vi "Launch On-Grid Optimization.vi"(8 "error in":errorcluster, 11 "SCADA in":refnum<class "EMS.lvclass">) -> (0 "error out":errorcluster, 3 "SCADA out":refnum<class "EMS.lvclass">)   [LabVIEW 2018, in "EMS Core.lvlib" / "EMS.lvclass"]
uses:
  EMS.lvclass
  C:/Users/Administrator/Desktop/LabVIEW EMS/EMS Generic Actor/EMS Generic/EMS Generic.lvclass
  C:/Program Files (x86)/National Instruments/LabVIEW 2018/vi.lib/ActorFramework/Actor/Actor.lvclass
  Optimization/On-Grid Actor/On-Grid/On-Grid.lvclass
  C:/Users/Administrator/Desktop/LabVIEW EMS/Device Communication and Control Abstract Actor/Device Communication and Control Abstract/Device Communication and Control Abstract.lvclass
  C:/Users/Administrator/Desktop/LabVIEW EMS/Optimization/Generic Optimization Actor/Generic Optimization/Generic Optimization.lvclass
  EMS Messages/Unintentional Island Occurence Msg/Unintentional Island Occurence Msg.lvclass
  C:/Users/Administrator/Desktop/LabVIEW EMS/Optimization/Generic Optimization Actor/Generic Optimization Messages/Operation Complete Msg/Operation Complete Msg.lvclass
  Optimization/Generic Optimization Actor/Generic Optimization/Generic Optimization.lvclass/Generic Optimization.ctl
  EMS.lvclass/EMS.ctl
  <vilib>/ActorFramework/Actor/Actor.lvclass
  Optimization/Generic Optimization Actor/Generic Optimization/Generic Optimization.lvclass
  Global Variables/Global Variables.vi
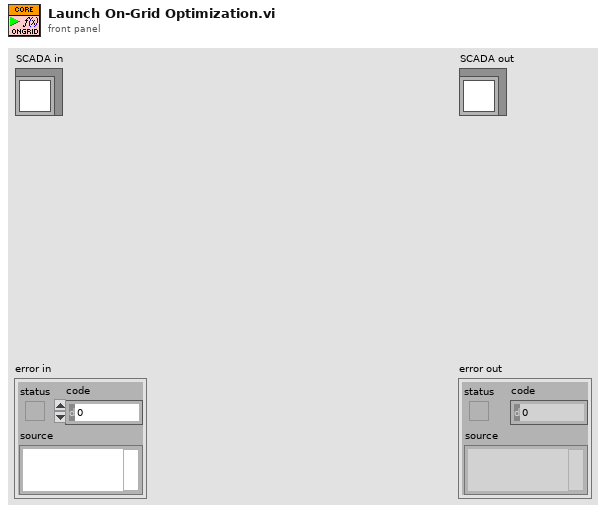
[diagram p1: front panel]
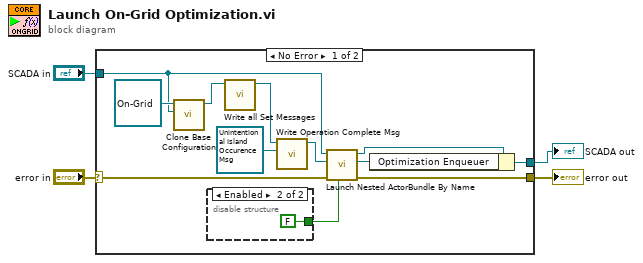
[diagram p0: block diagram]
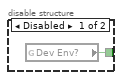
[diagram p2: hidden frame]
diagram:
  n1 = case shown="No Error" "error in" {
    selector: "error in" -> [w9 w20]
    tunnel: [w15 w20] -> w3
    tunnel: [w14 w19] -> w1
    tunnel: "SCADA in" -> [w6 w19]
    frame No Error {
      n2 = call-dynamic "Clone Base Configuration.vi"("Source Object"=w6, "Target Object in"=refnum<class "On-Grid.lvclass"> refnum ("On-Grid Actor.lvlib:On-Grid.lvclass")) -> ("Target Object out"=w7:refnum<class "On-Grid.lvclass">)  [unwired: 9 in]
      n3 = disable-structure shown="Enabled" {
        disable-tunnel: [w17 FALSE ("Open Actor Core front panel? (F)")] -> w5
        frame Disabled {
          n4 = global read "Global Variables.vi" "Dev Env?"() -> (w17:bool)
        }
        frame Enabled {
        }
      }
      n5 = call "Write all Set Messages.vi"("Device Communication and Control Abstract In"=w7) -> ("Device Communication and Control Abstract Out"=w12:refnum<class "On-Grid.lvclass">)  [unwired: 10 in]
      n6 = call "Write Operation Complete Msg.vi"("Operation Complete Msg"=refnum<class "Unintentional Island Occurence Msg.lvclass"> refnum ("SCADA Core.lvlib:Unintentional Island Occurence Msg.lvclass"), "Generic Optimization in"=w12) -> ("Generic Optimization out"=w11:refnum<class "On-Grid.lvclass">)  [unwired: 9 in]
      n7 = call <vilib>:"Launch Nested Actor.vi"("Open Actor Core front panel? (F)"=w5, "error in (no error)"=w9, "Nested Actor"=w11, "Caller Actor in"=w6) -> ("error out"=w15:errorcluster, "Nested Actor's Enqueuer"=w13:refnum<class "Message Enqueuer.lvclass">, "Caller Actor out"=w16:refnum<class "EMS.lvclass">)  [unwired: 5 in]
      n8 = Bundle By Name(cluster=w16, "Optimization Enqueuer"=w13) -> (w14:refnum<class "EMS.lvclass">)
    }
    frame Error {
    }
  }
  "error out" <- w3
  "SCADA out" <- w1
